vi "Untitled 4.vi"() -> ()   [LabVIEW 2015]
panel:
  out "key names":string[](array[string])
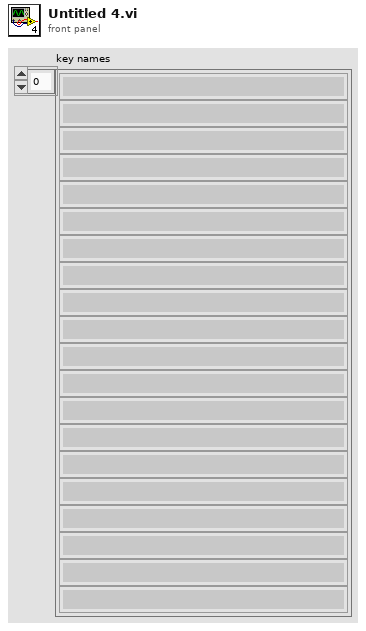
[diagram p1: front panel]
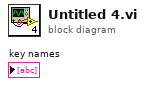
[diagram p0: block diagram]
diagram:
